vi "SetImageFormat.vi"(8 "error in (no error)":errorcluster caption="错误输入（无错误）", 10 "文件格式":T1(ring), 11 "Screen 输入":refnum<class "Screen.lvclass"> caption="DNL_LabVIEW Object in") -> (0 "error out":errorcluster caption="错误输出", 3 "Screen 输出":refnum<class "Screen.lvclass"> caption="DNL_LabVIEW Object out")   [LabVIEW 2011, in "Screen.lvclass"]
uses:
  Screen.lvclass
  Screen.lvclass/Screen.ctl
  System.Drawing
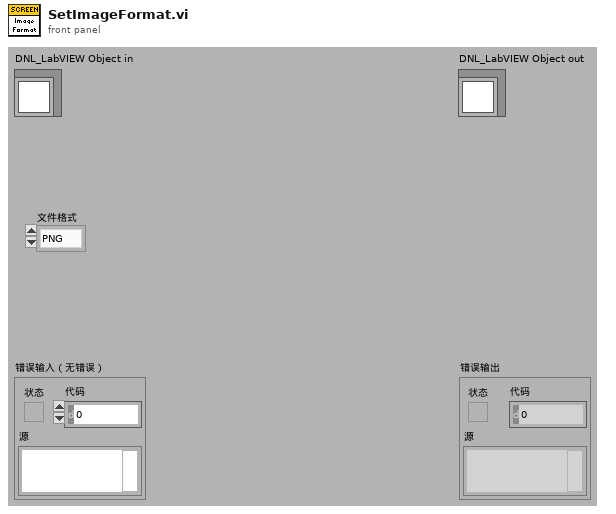
[diagram p1: front panel]
types:
  T1 = enum16{"PNG", "TIFF", "EMF", "JPEG", "BMP", "GIF"}
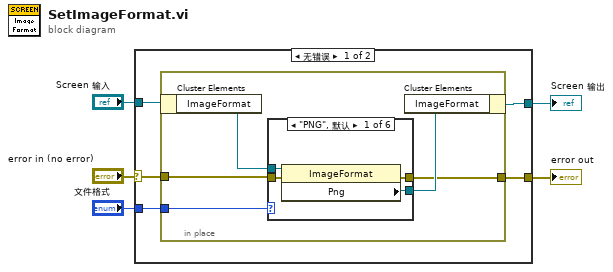
[diagram p0: block diagram]
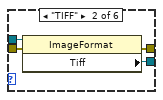
[diagram p2: hidden frame]
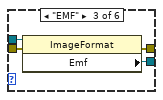
[diagram p3: hidden frame]
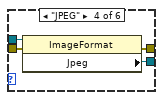
[diagram p4: hidden frame]
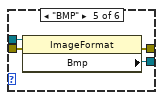
[diagram p5: hidden frame]
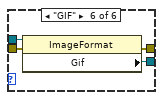
[diagram p6: hidden frame]
diagram:
  n1 = case shown="无错误" "error in (no error)" {
    selector: "error in (no error)" -> [w8 w41]
    tunnel: [w7 w41] -> w4
    tunnel: [w6 w40] -> w2
    tunnel: "Screen 输入" -> [w10 w40]
    tunnel: "文件格式" -> [w9 _]
    frame No Error {
      n2 = in-place {
        in-place-border: w9 -> [w15]
        in-place-border: w8 -> [w12]
        in-place-border: [w11] -> w7
        n3 = in-place-cluster #1(w10) -> ("ImageFormat"=w14:refnum<k24>)
        n4 = case shown="\"PNG\", 默认" w15 {
          tunnel: [w19 w23 w27 w31 w35 w39] -> w13
          tunnel: [w18 w22 w26 w30 w34 w38] -> w11
          tunnel: w14 -> [w17 w21 w25 w29 w33 w37]
          tunnel: w12 -> [w16 w20 w24 w28 w32 w36]
          frame "PNG", Default {
            n5 = property class="ImageFormat"(reference=w17, error in=w16) -> (error out=w18:errorcluster, "Png"=w19:refnum<k24>)  [unwired: 1 out]
          }
          frame "TIFF" {
            n6 = property class="ImageFormat"(reference=w21, error in=w20) -> (error out=w22:errorcluster, "Tiff"=w23:refnum<k24>)  [unwired: 1 out]
          }
          frame "EMF" {
            n7 = property class="ImageFormat"(reference=w25, error in=w24) -> (error out=w26:errorcluster, "Emf"=w27:refnum<k24>)  [unwired: 1 out]
          }
          frame "JPEG" {
            n8 = property class="ImageFormat"(reference=w29, error in=w28) -> (error out=w30:errorcluster, "Jpeg"=w31:refnum<k24>)  [unwired: 1 out]
          }
          frame "BMP" {
            n9 = property class="ImageFormat"(reference=w33, error in=w32) -> (error out=w34:errorcluster, "Bmp"=w35:refnum<k24>)  [unwired: 1 out]
          }
          frame "GIF" {
            n10 = property class="ImageFormat"(reference=w37, error in=w36) -> (error out=w38:errorcluster, "Gif"=w39:refnum<k24>)  [unwired: 1 out]
          }
        }
        n11 = in-place-cluster #1("ImageFormat"=w13) -> (w6:refnum<class "Screen.lvclass">)
      }
    }
    frame Error {
    }
  }
  "error out" <- w4
  "Screen 输出" <- w2
